vi "tabRef.vi"(8 "error in (no error)":errorcluster, 10 "control name":string, 11 "Tab Control":refnum<vi>) -> (0 "error out":errorcluster, 3 "control refnum":refnum<vi>)   [LabVIEW 2015]
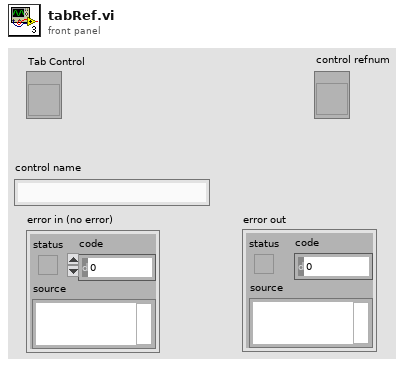
[diagram p1: front panel]
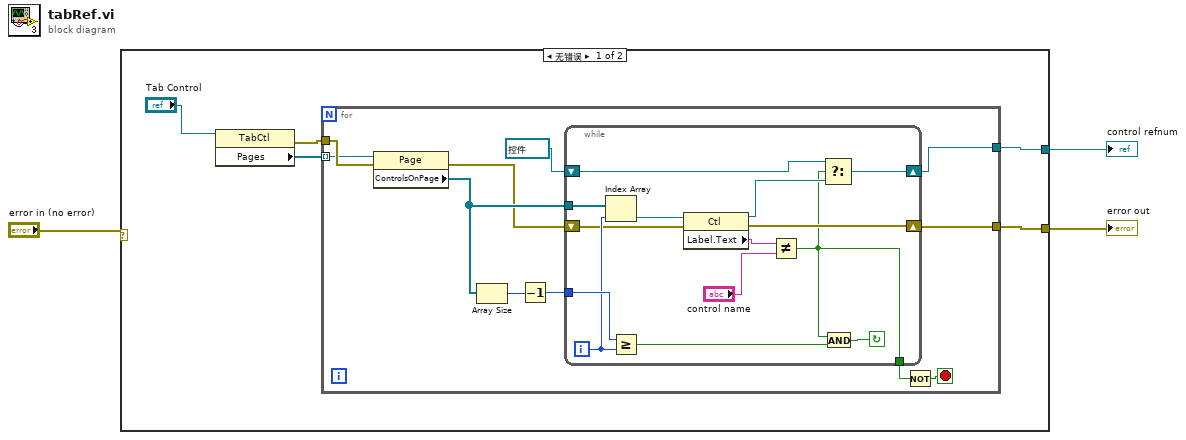
[diagram p0: block diagram]
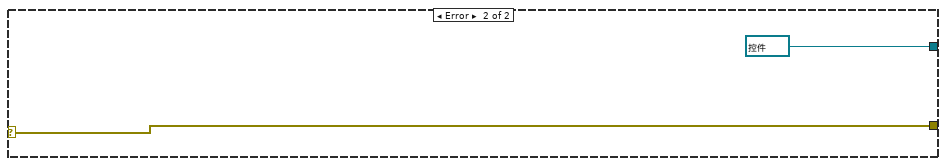
[diagram p2: hidden frame]
diagram:
  n1 = case shown="无错误" "error in (no error)" {
    selector: "error in (no error)" -> [_ w35]
    tunnel: [w6 refnum<vi> refnum ("dup reference")] -> w1
    tunnel: [w5 w35] -> w3
    frame No Error {
      n2 = property class="TabCtl"(reference="Tab Control") -> (error out=w8:errorcluster, "Pages"=w7:refnum<vi>[])  [unwired: 1 in, 1 out]
      n3 = for {
        tunnel: w8 -> [w19]
        tunnel: w7 -> [w18] mode=indexing
        tunnel: [w14] -> w6
        tunnel: [w11] -> w5
        stop <- w9 stop-if-true
        n4 = property class="Page"(reference=w18, error in=w19) -> (error out=w12:errorcluster, "ControlsOnPage"=w16:refnum<vi>[])  [unwired: 1 out]
        n5 = Array Size(array=w16) -> (size(s)=w17:i32)
        n6 = Decrement(x=w17) -> (x-1=w13:i32)
        n7 = while {
          tunnel: w13 -> [w33]
          tunnel: w16 -> [w32]
          shift-right: [w28] -> w14
          shift-left: refnum<vi> refnum ("dup reference") -> [w27]
          shift-right: [w23] -> w11
          shift-left: w12 -> [w24]
          tunnel: [w20] -> w10
          i -> [w31]
          stop <- w22 continue-if-true
          n8 = Index Array(array=w32, index=w31) -> (element=w30:refnum<vi>)
          n9 = Greater Or Equal?(x=w33, y=w31) -> (x >= y?=w25:bool)
          n10 = property class="Ctl"(reference=w30, error in=w24) -> (reference out=w26:refnum<vi>, error out=w23:errorcluster, "Label.Text"=w21:string)
          n11 = Not Equal?(x=w21, y="control name") -> (x != y?=w20:bool)
          n12 = Select(t=w27, s=w20, f=w26) -> (s? t:f=w28:refnum<vi>)
          n13 = And(x=w20, y=w25) -> (x .and. y?=w22:bool)
        }
        n14 = Not(x=w10) -> (.not. x?=w9:bool)
      }
    }
    frame Error {
    }
  }
  "control refnum" <- w1
  "error out" <- w3
